vi "Cluster.vi"(5 "模式 2":enum16{"select", "insert", "update", "delete"}(ring), 7 "productsName":string, 11 "limit":refnum<vi>) -> ()   [LabVIEW 2012]
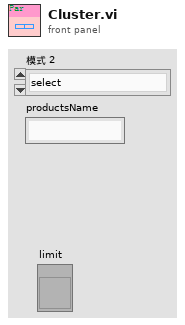
[diagram p1: front panel]
types:
  T1 = enum16{"selectdata", "selectsave", "selectlist", "selectshow"}
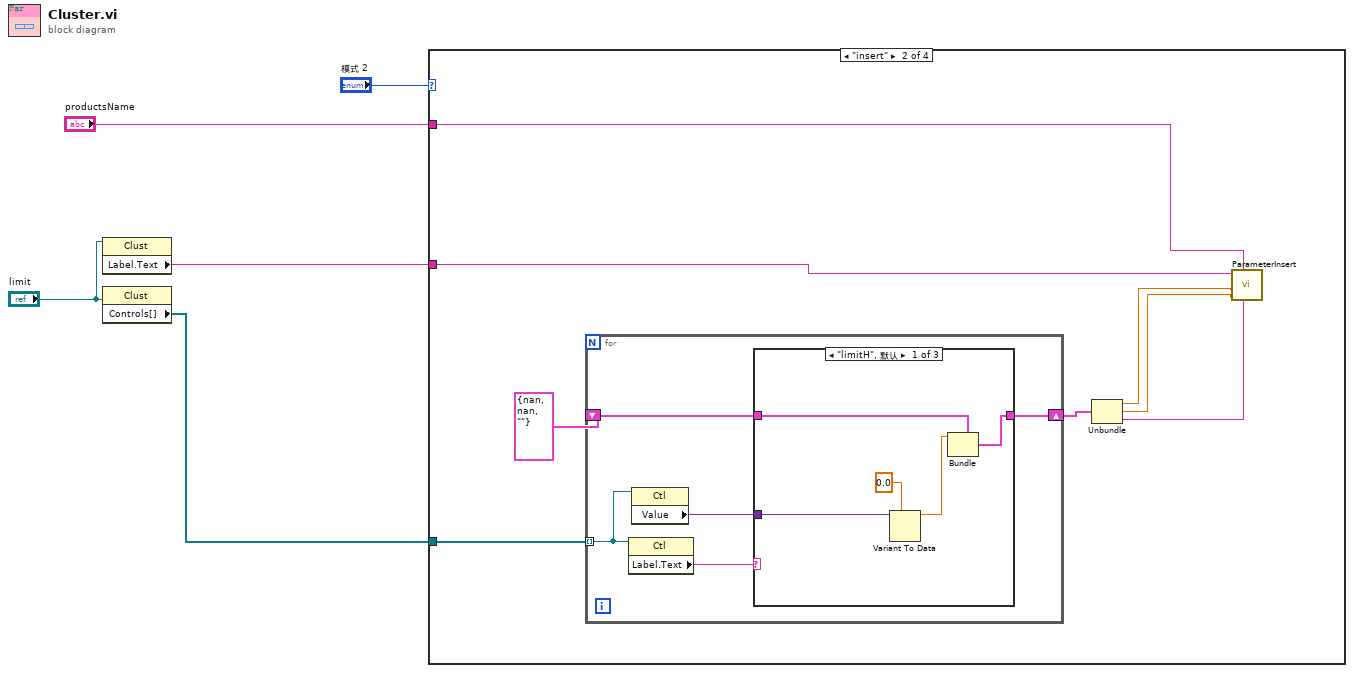
[diagram p0: block diagram]
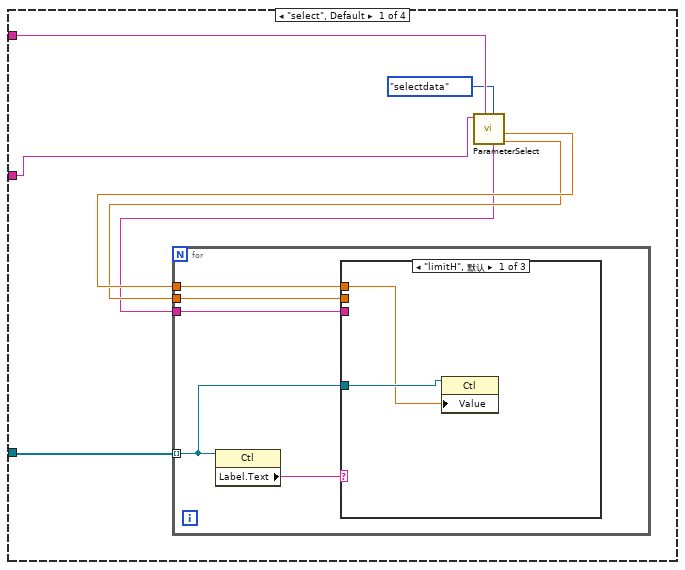
[diagram p2: hidden frame]
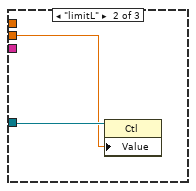
[diagram p3: hidden frame]
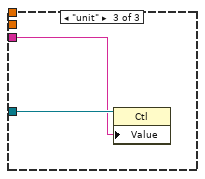
[diagram p4: hidden frame]
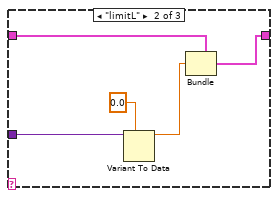
[diagram p5: hidden frame]
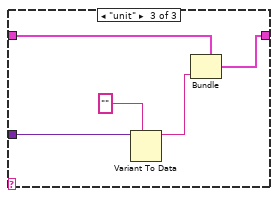
[diagram p6: hidden frame]
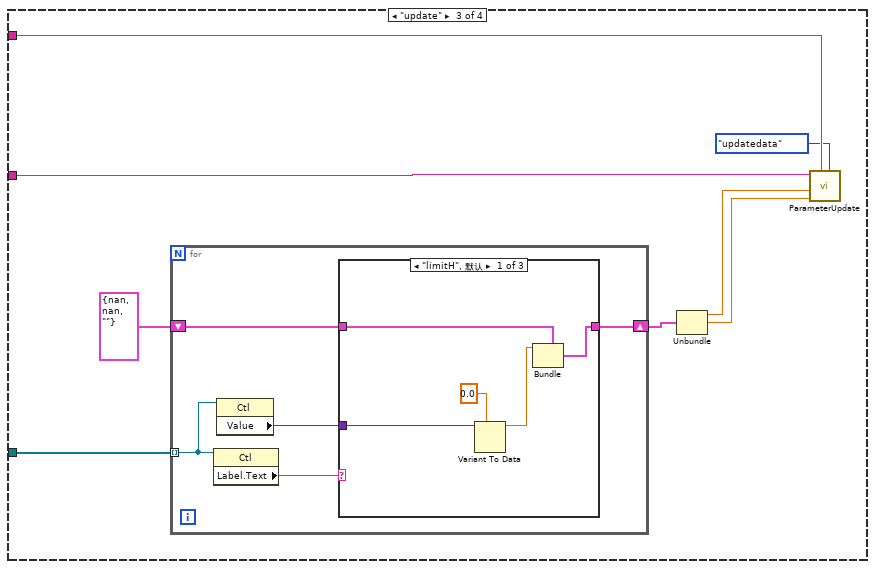
[diagram p7: hidden frame]
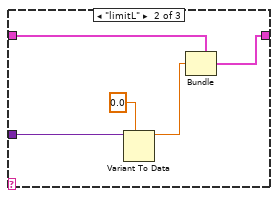
[diagram p8: hidden frame]
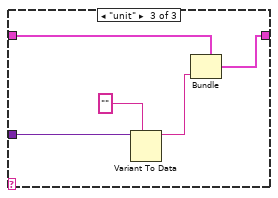
[diagram p9: hidden frame]
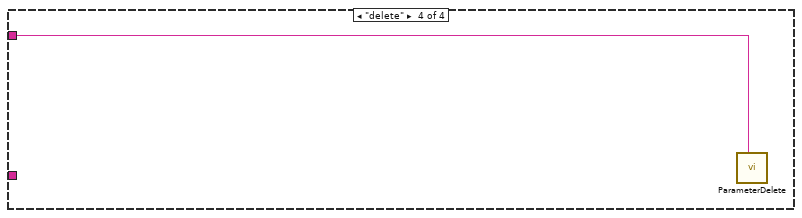
[diagram p10: hidden frame]
diagram:
  n1 = property on="属性节点" class="Clust"(reference="limit") -> ("Label.Text"=w3:string)  [unwired: 1 in, 2 out]
  n2 = property on="属性节点" class="Clust"(reference="limit") -> ("Controls[]"=w2:refnum<vi>[])  [unwired: 1 in, 2 out]
  n3 = case shown="\"insert\"" "模式 2" {
    tunnel: "productsName" -> [w11 w28 w56 w80]
    tunnel: w3 -> [w10 w27 w55 _]
    tunnel: w2 -> [w12 w30 w57 _]
    frame "select", Default {
      n4 = call "ParameterSelect.vi"("模式"=T1."selectdata", "productsName"=w11, "parameterName"=w10) -> ("limitL"=w8:dbl, "limitH"=w9:dbl, "unit"=w7:string)  [unwired: 3 in, 3 out]
      n5 = for {
        tunnel: w12 -> [w16] mode=indexing
        tunnel: w9 -> [w15]
        tunnel: w8 -> [w14]
        tunnel: w7 -> [w13]
        n6 = property on="属性节点" class="Ctl"(reference=w16) -> ("Label.Text"=w17:string)  [unwired: 1 in, 2 out]
        n7 = case shown="\"limitH\", 默认" w17 {
          tunnel: w16 -> [w19 w21 w23]
          tunnel: w15 -> [w18 _ _]
          tunnel: w14 -> [_ w20 _]
          tunnel: w13 -> [_ _ w22]
          frame "limitH", Default {
            n8 = property on="属性节点" class="Ctl"(reference=w19, "Value"=w18) -> ()  [unwired: 1 in, 2 out]
          }
          frame "limitL" {
            n9 = property on="属性节点" class="Ctl"(reference=w21, "Value"=w20) -> ()  [unwired: 1 in, 2 out]
          }
          frame "unit" {
            n10 = property on="属性节点" class="Ctl"(reference=w23, "Value"=w22) -> ()  [unwired: 1 in, 2 out]
          }
        }
      }
    }
    frame "insert" {
      n11 = for {
        tunnel: w30 -> [w33] mode=indexing
        shift-right: [w34] -> w29
        shift-left: cluster{"vaule":dbl, "vaule":dbl, "说明信息":string} {"vaule"=nan, "vaule"=nan, "说明信息"=""} ("输出簇") -> [w35]
        n12 = property on="属性节点" class="Ctl"(reference=w33) -> ("Label.Text"=w36:string)  [unwired: 1 in, 2 out]
        n13 = property on="属性节点" class="Ctl"(reference=w33) -> ("Value"=w32:variant)  [unwired: 1 in, 2 out]
        n14 = case shown="\"limitH\", 默认" w36 {
          tunnel: w35 -> [w40 w44 w49]
          tunnel: [w39 w43 w48] -> w34
          tunnel: w32 -> [w38 w45 w50]
          frame "limitH", Default {
            n15 = Variant To Data(type=0.0 ("vaule"), Variant=w38) -> (data=w37:dbl)  [unwired: 1 in, 1 out]
            n16 = Bundle(cluster=w40, "vaule"=w37) -> (w39:cluster{"vaule":dbl, "vaule":dbl, "说明信息":string})  [unwired: 2 in]
          }
          frame "limitL" {
            n17 = Variant To Data(type=0.0 ("vaule"), Variant=w45) -> (data=w42:dbl)  [unwired: 1 in, 1 out]
            n18 = Bundle(cluster=w44, "vaule"=w42) -> (w43:cluster{"vaule":dbl, "vaule":dbl, "说明信息":string})  [unwired: 2 in]
          }
          frame "unit" {
            n19 = Variant To Data(type="" ("说明信息"), Variant=w50) -> (data=w47:string)  [unwired: 1 in, 1 out]
            n20 = Bundle(cluster=w49, "说明信息"=w47) -> (w48:cluster{"vaule":dbl, "vaule":dbl, "说明信息":string})  [unwired: 2 in]
          }
        }
      }
      n21 = Unbundle(w29) -> ("vaule"=w26:dbl, "vaule"=w25:dbl, "说明信息"=w24:string)
      n22 = call "ParameterInsert.vi"("unit"=w24, "productsName"=w28, "limitL"=w25, "limitH"=w26, "parameterName"=w27) -> ()  [unwired: 7 in]
    }
    frame "update" {
      n23 = for {
        tunnel: w57 -> [w61] mode=indexing
        shift-right: [w62] -> w58
        shift-left: cluster{"vaule":dbl, "vaule":dbl, "说明信息":string} {"vaule"=nan, "vaule"=nan, "说明信息"=""} ("输出簇") -> [w63]
        n24 = property on="属性节点" class="Ctl"(reference=w61) -> ("Label.Text"=w64:string)  [unwired: 1 in, 2 out]
        n25 = property on="属性节点" class="Ctl"(reference=w61) -> ("Value"=w60:variant)  [unwired: 1 in, 2 out]
        n26 = case shown="\"limitH\", 默认" w64 {
          tunnel: w63 -> [w68 w72 w77]
          tunnel: [w67 w71 w76] -> w62
          tunnel: w60 -> [w66 w73 w78]
          frame "limitH", Default {
            n27 = Variant To Data(type=0.0 ("vaule"), Variant=w66) -> (data=w65:dbl)  [unwired: 1 in, 1 out]
            n28 = Bundle(cluster=w68, "vaule"=w65) -> (w67:cluster{"vaule":dbl, "vaule":dbl, "说明信息":string})  [unwired: 2 in]
          }
          frame "limitL" {
            n29 = Variant To Data(type=0.0 ("vaule"), Variant=w73) -> (data=w70:dbl)  [unwired: 1 in, 1 out]
            n30 = Bundle(cluster=w72, "vaule"=w70) -> (w71:cluster{"vaule":dbl, "vaule":dbl, "说明信息":string})  [unwired: 2 in]
          }
          frame "unit" {
            n31 = Variant To Data(type="" ("说明信息"), Variant=w78) -> (data=w75:string)  [unwired: 1 in, 1 out]
            n32 = Bundle(cluster=w77, "说明信息"=w75) -> (w76:cluster{"vaule":dbl, "vaule":dbl, "说明信息":string})  [unwired: 2 in]
          }
        }
      }
      n33 = Unbundle(w58) -> ("vaule"=w53:dbl, "vaule"=w52:dbl)  [unwired: 1 out]
      n34 = call "ParameterUpdate.vi"("模式"=enum16{"updatedata", "updatesave"}."updatedata", "productsName"=w56, "limitL"=w52, "limitH"=w53, "parameterName"=w55) -> ()  [unwired: 7 in]
    }
    frame "delete" {
      n35 = call "ParameterDelete.vi"("productsName"=w80) -> ()  [unwired: 11 in]
    }
  }
